vi "CHEMPOTdll.vi"(8 "error in (no error)":errorcluster, 11 "Inputs":cluster{"t":dbl, "D":dbl, "z":dbl[]}) -> (0 "error out":errorcluster, 3 "Outputs":T1)   [LabVIEW 2016]
doc: "subroutine CHEMPOTdll(t, d, z, u, ierr, herr, herr_length)\nCompute the chemical potentials for each of the nc components of a mixture.\n\nINPUTS:\nt -- Temperature [K]\nD -- Molar density [mol/L]\nz -- Composition (array of mole fractions)\n\nOUTPUTS:\nu -- Array (1..nc) of the chemical potentials [J/mol]\nierr -- error flag: 0 = successful\nherr -- error string\nherr_length -- length of variable herr (default: 255)"
uses:
  REFPROP.DLL
panel:
  # "REFPROP-CHEMPOTdll.vi"
  # "void  CHEMPOTdll(double *t, double *D, double *z, double *u, int32_t *ierr, CStr herr, int32_t herr_length)"
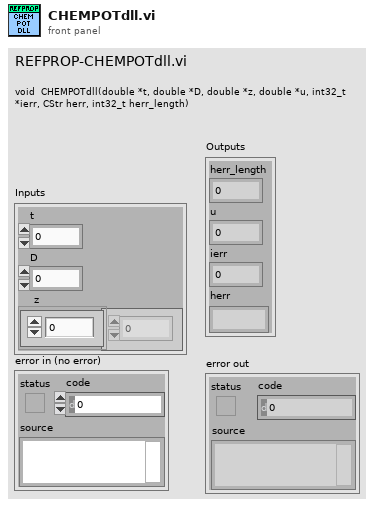
[diagram p1: front panel]
types:
  T1 = cluster{"u":dbl, "ierr":i32, "herr":string, "herr_length":i32}
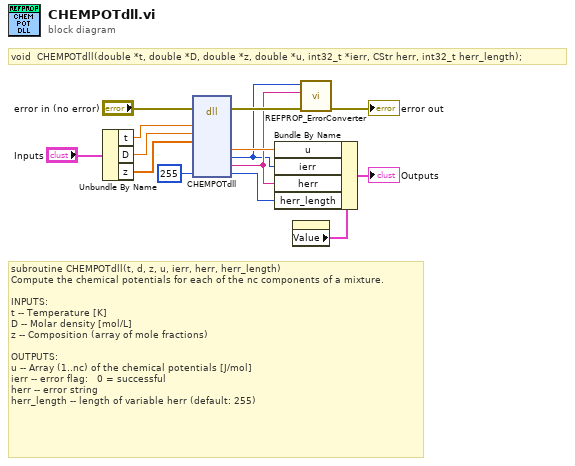
[diagram p0: block diagram]
diagram:
  # "void  CHEMPOTdll(double *t, double *D, double *z, double *u, int32_t *ierr, CStr herr, int32_t herr_length);"
  # "subroutine CHEMPOTdll(t, d, z, u, ierr, herr, herr_length)\nCompute the chemical potentials for each of the nc components of a mixture.\n\nINPUTS:\nt -- Temperature [K]\nD -- Molar density [mol/L]\nz -- Composition (array of mole fractions)\n\nOUTPUTS:\nu -- Array (1..nc) of the chemical potentials [J/mol]\nierr -- error flag:   0 = successful\nherr -- error string\nherr_length -- length of variable herr (default: 255)"
  n1 = Unbundle By Name("Inputs") -> ("t"=w9:dbl, "D"=w8:dbl, "z"=w7:dbl[])
  n2 = dll-call lib="S:/009 - Testing/02 - Performance Testing/REFPROP/REFPROP.*" fn="CHEMPOTdll"(error in="error in (no error)", "t"=w9, "D"=w8, "z"=w7, "herr_length"=255 ("ln")) -> (error out=w13:errorcluster, "u"=w3:dbl, "ierr"=w1:i32, "herr"=w2:string, "herr_length"=w4:i32)  [unwired: 9 in, 1 out]
  n3 = property on="Outputs" class="Clust (strict)"() -> ("Value"=w6:T1)  [unwired: 2 in, 2 out]
  n4 = Bundle By Name(cluster=w6, "u"=w3, "ierr"=w1, "herr"=w2, "herr_length"=w4) -> (→"Outputs":T1)
  n5 = call "REFPROP_ErrorConverter.vi"("error in (no error)"=w13, "Error Message"=w2, "Error Code"=w1) -> ("error out"=→"error out":errorcluster)  [unwired: 8 in]
